vi "String to Numeric Array.vi"(10 "String Array":string[](array[string])) -> (2 "Numeric Array":dbl[](array[numeric]))   [LabVIEW 2013, in "Keithley 27XX.lvlib"]
doc: "Use this VI to convert an array of strings to numeric where applicable in driver. For example, converting the timestamp array to an array of numerics."
uses:
  <instrlib>/Keithley 27XX/Keithley 27XX.lvlib
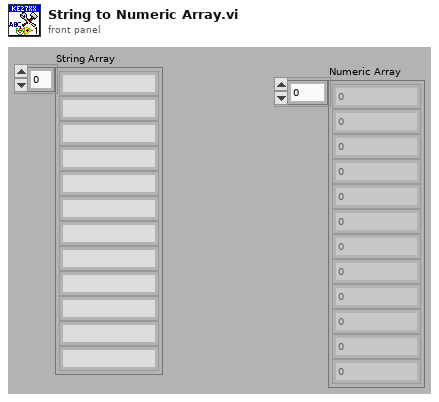
[diagram p1: front panel]
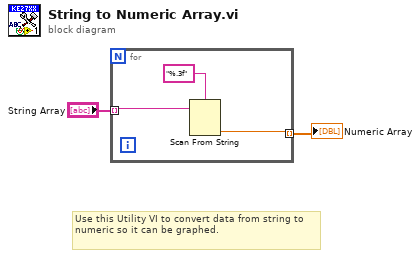
[diagram p0: block diagram]
diagram:
  # "Use this Utility VI to convert data from string to numeric so it can be graphed."
  n1 = for {
    tunnel: "String Array" -> [w5] mode=indexing
    tunnel: [w3] -> w1 mode=indexing
    n2 = Scan From String(format string="%.3f", input string=w5) -> (output 1=w3:dbl)  [unwired: 3 in, 3 out]
  }
  "Numeric Array" <- w1
